vi "WriteLog.vi"(1 "String":string) -> ()   [LabVIEW 2021]
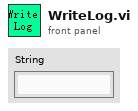
[diagram p1: front panel]
types:
  T1 = enum16{"open", "replace", "create", "open or create", "replace or create", "replace or create with confirmation"}
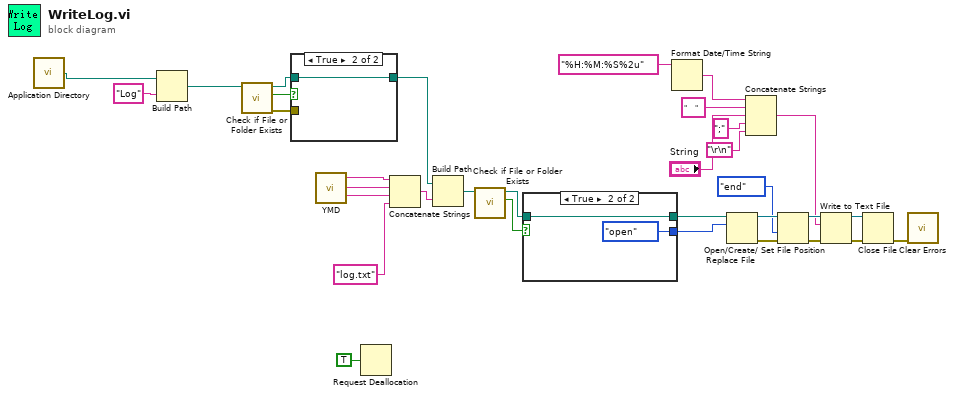
[diagram p0: block diagram]
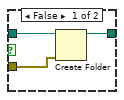
[diagram p2: hidden frame]
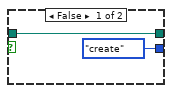
[diagram p3: hidden frame]
diagram:
  n1 = call <vilib>:"Application Directory.vi"() -> ("Application Directory"=w1:path)
  n2 = Build Path(base path=w1, name or relative path="Log") -> (appended path=w11:path)
  n3 = call <vilib>:"Check if File or Folder Exists.vi"("path"=w11) -> ("error out"=w8:errorcluster, "file or folder exists?"=w10:bool, "dup path"=w9:path)  [unwired: 8 in]
  n4 = case shown="True" w10 {
    tunnel: w9 -> [w36 w37]
    tunnel: w8 -> [w35 _]
    tunnel: [w34 w37] -> w7
    frame False {
      n5 = Create Folder(path (use dialog)=w36, error in=w35) -> (created path=w34:path)  [unwired: 1 in, 2 out]
    }
    frame True {
    }
  }
  n6 = call "YMD.vi"() -> ("DD"=w3:string, "MM"=w4:string, "YYYY"=w5:string)
  n7 = Request Deallocation(TRUE ("flag")) -> ()
  n8 = Concatenate Strings(w5, w4, w3, "log.txt" ("string")) -> (w18:string)
  n9 = Build Path(base path=w7, name or relative path=w18) -> (appended path=w17:path)
  n10 = call <vilib>:"Check if File or Folder Exists.vi"("path"=w17) -> ("file or folder exists?"=w16:bool, "dup path"=w15:path)  [unwired: 8 in, 1 out]
  n11 = case shown="True" w16 {
    tunnel: w15 -> [w39 w41]
    tunnel: [w39 w41] -> w28
    tunnel: [T1."create" ("operation (0:open)") T1."open" ("operation (0:open)")] -> w14
    frame False {
    }
    frame True {
    }
  }
  n12 = Format Date/Time String(time format string (%c)="%H:%M:%S%2u") -> (date/time string=w32:string)  [unwired: 2 in]
  n13 = Open/Create/Replace File(file path (use dialog)=w28, operation (0:open)=w14) -> (refnum out=w27:refnum<file>, error out=w26:errorcluster)  [unwired: 4 in, 1 out]
  n14 = Concatenate Strings(w32, "    " ("string"), "String", ";" ("string"), "\r\n") -> (w22:string)
  n15 = Set File Position(refnum=w27, from (0:start)=enum16{"start", "end", "current"}."end", error in=w26) -> (refnum out=w24:refnum<file>, error out=w25:errorcluster)  [unwired: 1 in]
  n16 = Write to Text File(file (use dialog)=w24, text=w22, error in=w25) -> (refnum out=w21:refnum<file>, error out=w20:errorcluster)  [unwired: 1 in, 1 out]
  n17 = Close File(refnum=w21, error in=w20) -> (error out=w2:errorcluster)  [unwired: 1 out]
  n18 = call <vilib>:"Clear Errors.vi"("error in (no error)"=w2) -> ()  [unwired: 5 in, 2 out]
